vi "SetParametersAndor.vi"(6 "Error In":errorcluster, 8 "Camera Information":T7 {"VS Speed (us)" format="%.2f"}, 9 "Andor Initialization Error Codes":T6, 10 "Acquisition Parameters":T3={"Acquisition Mode"=enum."Single Scan", "Trigger Mode"=enum."Internal", "Frame \nTransfer"=FALSE, "Exposure Time (s)"=0.0, "Accumulation Cycle Time (s)"=0.0, "# Accumulations"=1, "# Kinetics"=1, "Kinetic Cycle Time (s)"=0.0, "Horizontal Bin Size"=1, "Vertical Bin Size"=1} {"Vertical Bin Size" min=1; "Horizontal Bin Size" min=1; "Kinetic Cycle Time (s)" format="%.2f"; "# Kinetics" min=1; "# Accumulations" min=1; "Accumulation Cycle Time (s)" format="%.2f"; "Exposure Time (s)" format="%.2f"}, 11 "Pre Initialized?":bool) -> (0 "error out":errorcluster, 2 "Calcualted Times":T1 {"Kinetic" format="%.4f"; "Accumulate" format="%.4f"; "Exposure" format="%.4f"}, 3 "Acq. Error Codes":T2)   [LabVIEW 2013]
uses:
  camera_information.ctl
  camera_controls.ctl
  <userlib>/atmcd32d.llb/AcquisitionMode_mode typedef.ctl
  <userlib>/atmcd32d.llb/TriggerMode_mode typedef.ctl
  set_parameters_states.ctl
  <userlib>/atmcd32d.llb/ReadMode_mode typedef.ctl
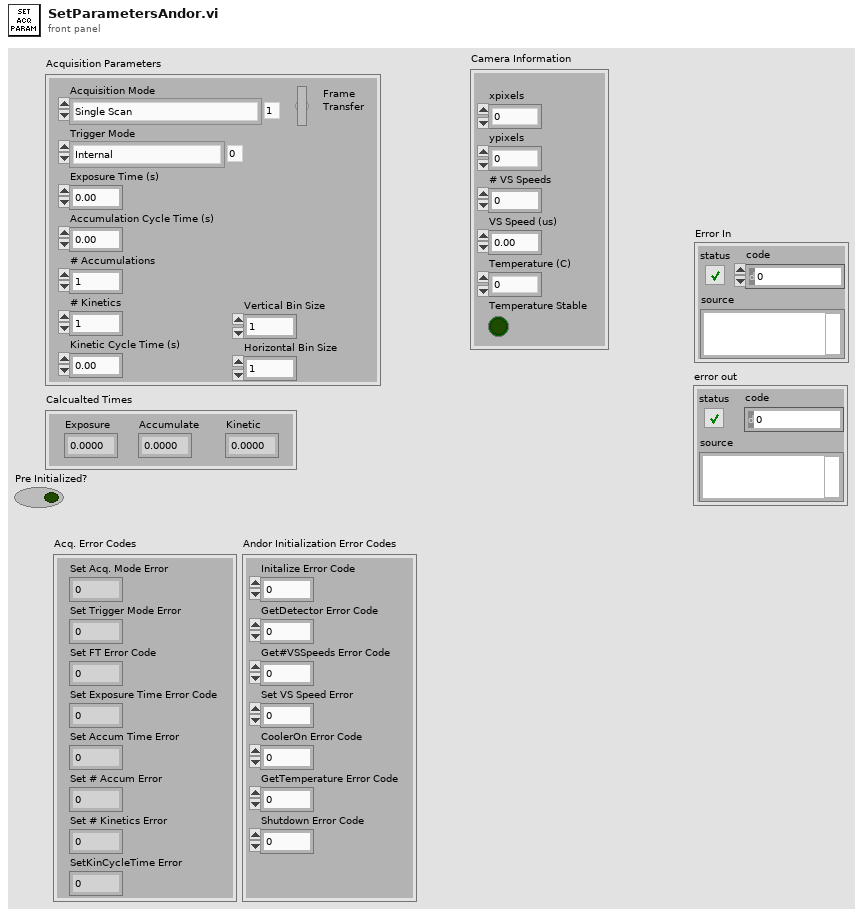
[diagram p1: front panel]
types:
  T1 = cluster{"Exposure":sgl, "Accumulate":sgl, "Kinetic":sgl}
  T2 = cluster{"Set Acq. Mode Error":u32, "Set Trigger Mode Error":u32, "Set FT Error Code":u32, "Set Exposure Time Error Code":u32, "Set Accum Time Error":u32, "Set # Accum Error":u32, "Set # Kinetics Error":u32, "SetKinCycleTime Error":u32}
  T3 = typedef "camera_controls.ctl" = cluster{"Acquisition Mode":T4, "Trigger Mode":T5, "Frame \nTransfer":bool, "Exposure Time (s)":sgl, "Accumulation Cycle Time (s)":sgl, "# Accumulations":i32, "# Kinetics":i32, "Kinetic Cycle Time (s)":sgl, "Horizontal Bin Size":i32, "Vertical Bin Size":i32}
  T4 = typedef "AcquisitionMode_mode typedef.ctl" = enum16{"Reserved (0)", "Single Scan", "Accumulate", "Kinetics", "Fast Kinetics", "Run Till Abort", "Reserved (6)", "Reserved (7)", "Reserved (8)", "Time Delayed Integration"}
  T5 = typedef "TriggerMode_mode typedef.ctl" = enum16{"Internal", "External", "N/A (2)", "N/A (3)", "N/A (4)", "N/A (5)", "External Start", "External Exposure (Bulb)", "N/A (8)", "External FVB EM", "Software", "N/A (11)", "External Charge Shifting"}
  T6 = cluster{"Initalize Error Code":u32, "GetDetector Error Code":u32, "Get#VSSpeeds Error Code":u32, "Set VS Speed Error":u32, "CoolerOn Error Code":u32, "GetTemperature Error Code":u32, "Shutdown Error Code":u32}
  T7 = typedef "camera_information.ctl" = cluster{"xpixels":i32, "ypixels":i32, "# VS Speeds":i32, "VS Speed (us)":sgl, "Temperature Stable":bool, "Temperature (C)":i32}
  T8 = typedef "set_parameters_states.ctl" = enum16{"Initialize", "Set Acq. Parameters", "Set Acq. Parameters 2", "Calculate", "Close Without Error", "Shutdown"}
  T9 = typedef "ReadMode_mode typedef.ctl" = enum16{"Full Vertical Binning", "Multi-Track", "Random-Track", "Single-Track", "Image"}
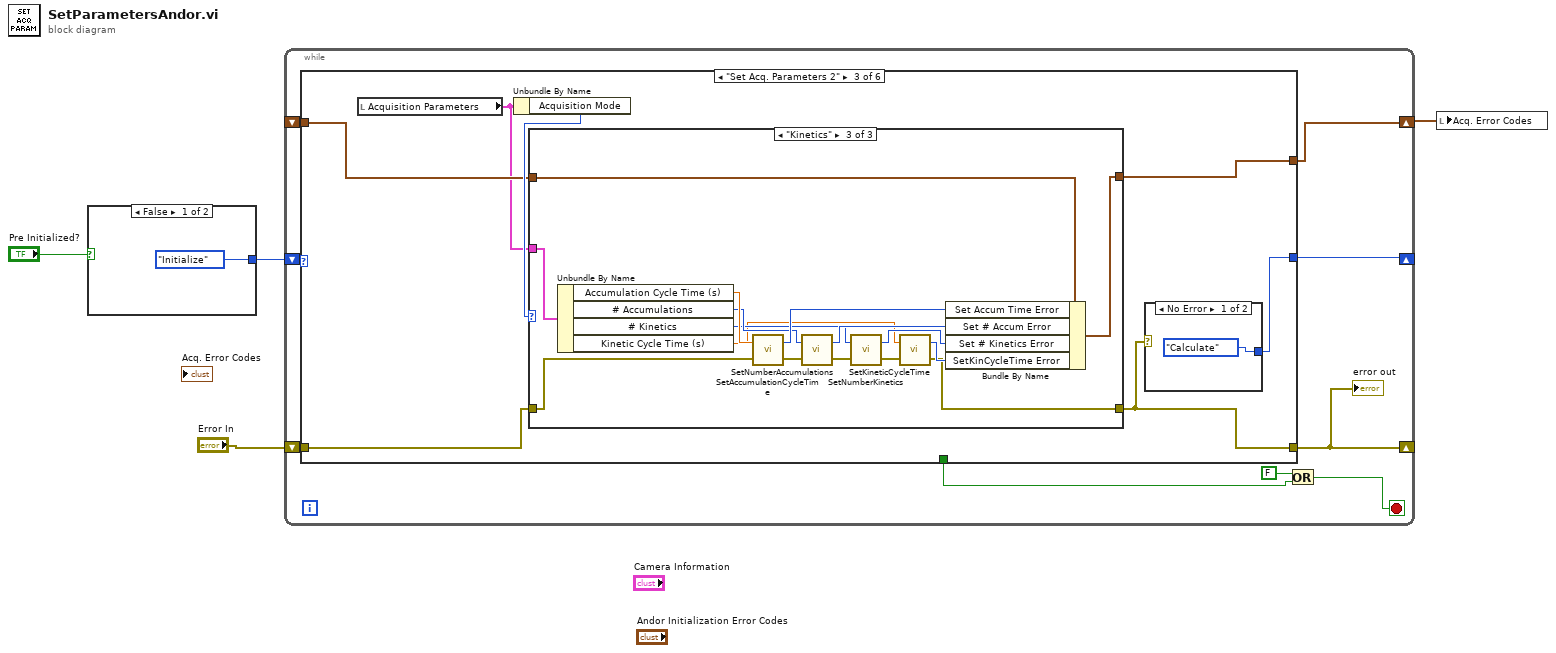
[diagram p0: block diagram]
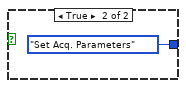
[diagram p2: hidden frame]
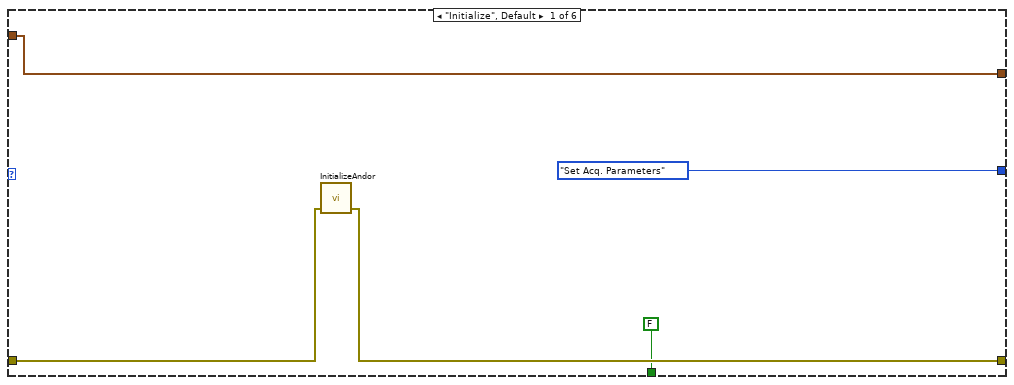
[diagram p3: hidden frame]
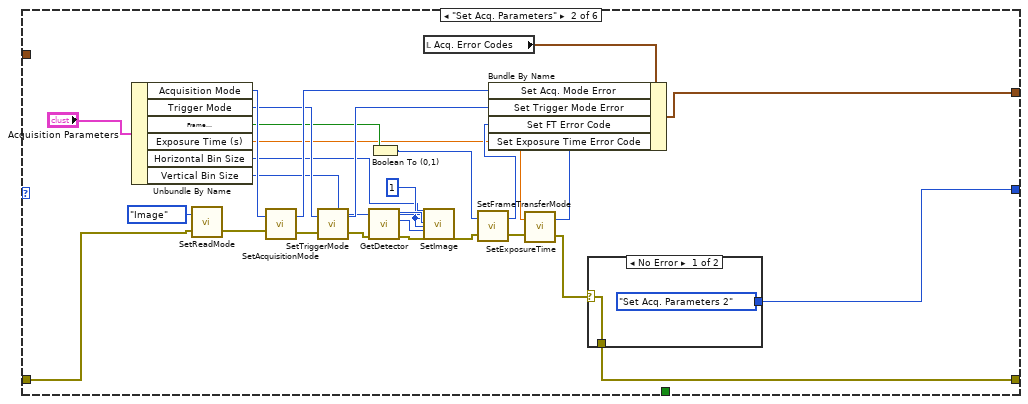
[diagram p4: hidden frame]
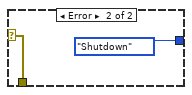
[diagram p5: hidden frame]
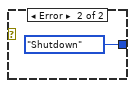
[diagram p6: hidden frame]
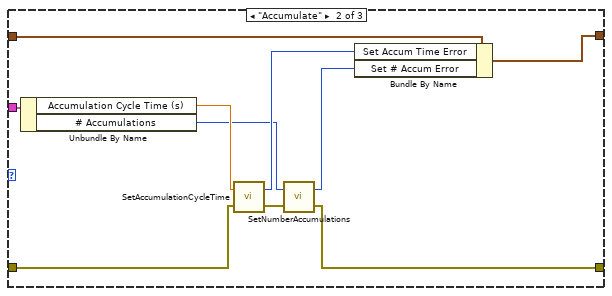
[diagram p8: hidden frame]
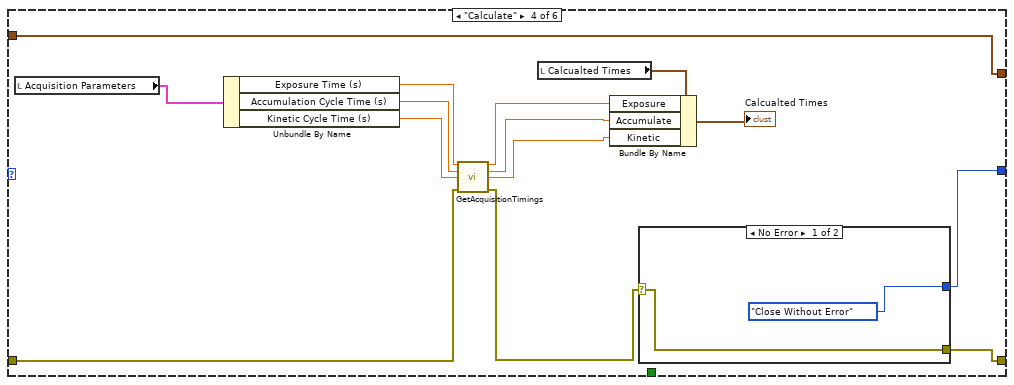
[diagram p9: hidden frame]
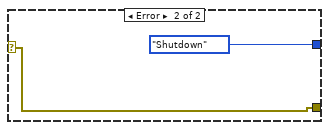
[diagram p10: hidden frame]
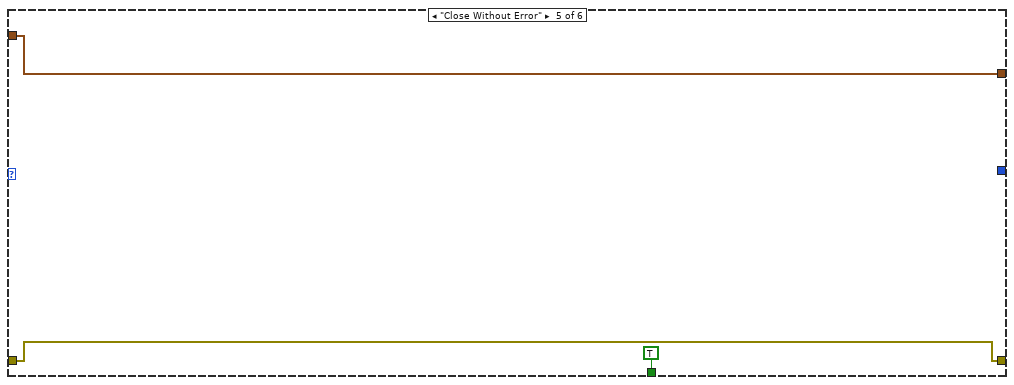
[diagram p11: hidden frame]
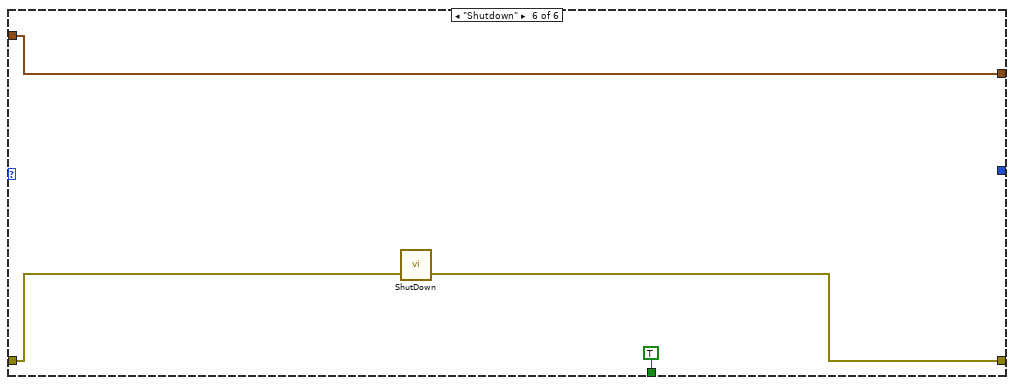
[diagram p12: hidden frame]
diagram:
  n1 = case shown="False" "Pre Initialized?" {
    tunnel: [set_parameters_states."Initialize" set_parameters_states."Set Acq. Parameters"] -> w4
    frame False {
    }
    frame True {
    }
  }
  n2 = while {
    shift-right: [w11] -> _
    shift-left: "Error In" -> [w14]
    shift-right: [w13] -> _
    shift-left: w4 -> [w15]
    shift-right: [w12] -> w2
    shift-left: _ -> [w7]
    stop <- w10 stop-if-true
    n3 = case shown="\"Set Acq. Parameters 2\"" w15 {
      tunnel: w14 -> [w20 w24 w58 w103 w109 w114]
      tunnel: [w19 w27 w54 w92 w109 w113] -> w11
      tunnel: [set_parameters_states."Set Acq. Parameters" w26 w53 w91 _ _] -> w13
      tunnel: [w16 w46 w55 w90 w108 w111] -> w12
      tunnel: [FALSE _ _ _ TRUE TRUE] -> w9
      tunnel: w7 -> [w16 _ w57 w90 w108 w111]
      frame "Initialize", Default {
        n4 = call "InitializeAndor.vi"("Error In"=w20) -> ("error out"=w19:errorcluster)  [unwired: 2 in, 2 out]
      }
      frame "Set Acq. Parameters" {
        w38 = 1
        n5 = Unbundle By Name("Acquisition Parameters") -> ("Acquisition Mode"=w44:T4, "Trigger Mode"=w42:T5, "Frame \nTransfer"=w34:bool, "Exposure Time (s)"=w31:sgl, "Horizontal Bin Size"=w21:i32, "Vertical Bin Size"=w22:i32)
        n6 = call <userlib>:"SetReadMode.vi"("error in (no error)"=w24, "mode"=ReadMode_mode_typedef."Image") -> ("error out"=w25:errorcluster)  [unwired: 1 out]
        n7 = call <userlib>:"SetAcquisitionMode.vi"("error in (no error)"=w25, "mode"=w44) -> ("error out"=w43:errorcluster, "DLL error code"=w47:u32)
        n8 = call <userlib>:"SetTriggerMode.vi"("error in (no error)"=w43, "mode"=w42) -> ("error out"=w36:errorcluster, "DLL error code"=w41:u32)
        n9 = call <userlib>:"GetDetector.vi"("error in (no error)"=w36) -> ("error out"=w40:errorcluster, "ypixels"=w37:i32, "xpixels"=w39:i32)  [unwired: 3 in, 1 out]
        n10 = Boolean To (0,1)(Boolean=w34) -> (0, 1=w33:i16)
        n11 = local read "Acq. Error Codes"() -> (w48:T2)
        n12 = call "SetImage.vi"("hbin"=w21, "vbin"=w22, "hstart"=w38, "hend"=w39, "vstart"=w38, "vend"=w37, "error in (no error)"=w40) -> ("error out"=w35:errorcluster)  [unwired: 19 in, 1 out]
        n13 = call <userlib>:"SetFrameTransferMode.vi"("error in (no error)"=w35, "mode"=w33) -> ("error out"=w29:errorcluster, "DLL error code"=w32:u32)
        n14 = call <userlib>:"SetExposureTime.vi"("error in (no error)"=w29, "time"=w31) -> ("error out"=w28:errorcluster, "DLL error code"=w30:u32)
        n15 = Bundle By Name(cluster=w48, "Set Acq. Mode Error"=w47, "Set Trigger Mode Error"=w41, "Set FT Error Code"=w32, "Set Exposure Time Error Code"=w30) -> (w46:T2)
        n16 = case shown="No Error" w28 {
          selector: w28 -> [w50 w51]
          tunnel: [w50 w51] -> w27
          tunnel: [set_parameters_states."Set Acq. Parameters 2" set_parameters_states."Shutdown"] -> w26
          frame No Error {
          }
          frame Error {
          }
        }
      }
      frame "Set Acq. Parameters 2" {
        n17 = local read "Acquisition Parameters"() -> (w56:T3)
        n18 = Unbundle By Name(w56) -> ("Acquisition Mode"=w59:T4)
        n19 = case shown="\"Kinetics\"" w59 {
          tunnel: [w63 w64 w74] -> w54
          tunnel: w58 -> [w63 w73 w89]
          tunnel: w57 -> [w62 w70 w87]
          tunnel: w56 -> [_ w72 w83]
          tunnel: [w62 w68 w84] -> w55
          frame "Single Scan", Default {
          }
          frame "Accumulate" {
            n20 = Unbundle By Name(w72) -> ("Accumulation Cycle Time (s)"=w71:sgl, "# Accumulations"=w66:i32)
            n21 = call <userlib>:"SetAccumulationCycleTime.vi"("error in (no error)"=w73, "time"=w71) -> ("error out"=w67:errorcluster, "DLL error code"=w69:u32)
            n22 = call <userlib>:"SetNumberAccumulations.vi"("error in (no error)"=w67, "number"=w66) -> ("error out"=w64:errorcluster, "DLL error code"=w65:u32)
            n23 = Bundle By Name(cluster=w70, "Set Accum Time Error"=w69, "Set # Accum Error"=w65) -> (w68:T2)
          }
          frame "Kinetics" {
            n24 = Unbundle By Name(w83) -> ("Accumulation Cycle Time (s)"=w82:sgl, "# Accumulations"=w81:i32, "# Kinetics"=w78:i32, "Kinetic Cycle Time (s)"=w76:sgl)
            n25 = call <userlib>:"SetAccumulationCycleTime.vi"("error in (no error)"=w89, "time"=w82) -> ("error out"=w88:errorcluster, "DLL error code"=w86:u32)
            n26 = call <userlib>:"SetNumberAccumulations.vi"("error in (no error)"=w88, "number"=w81) -> ("error out"=w80:errorcluster, "DLL error code"=w85:u32)
            n27 = call <userlib>:"SetNumberKinetics.vi"("error in (no error)"=w80, "number"=w78) -> ("error out"=w77:errorcluster, "DLL error code"=w79:u32)
            n28 = call <userlib>:"SetKineticCycleTime.vi"("error in (no error)"=w77, "time"=w76) -> ("error out"=w74:errorcluster, "DLL error code"=w75:u32)
            n29 = Bundle By Name(cluster=w87, "Set Accum Time Error"=w86, "Set # Accum Error"=w85, "Set # Kinetics Error"=w79, "SetKinCycleTime Error"=w75) -> (w84:T2)
          }
        }
        n30 = case shown="No Error" w54 {
          tunnel: [set_parameters_states."Calculate" set_parameters_states."Shutdown"] -> w53
          frame No Error {
          }
          frame Error {
          }
        }
      }
      frame "Calculate" {
        n31 = local read "Acquisition Parameters"() -> (w102:T3)
        n32 = Unbundle By Name(w102) -> ("Exposure Time (s)"=w101:sgl, "Accumulation Cycle Time (s)"=w100:sgl, "Kinetic Cycle Time (s)"=w99:sgl)
        n33 = call <userlib>:"GetAcquisitionTimings.vi"("exposure input"=w101, "accumulate input"=w100, "kinetic input"=w99, "error in (no error)"=w103) -> ("exposure"=w97:sgl, "accumulate"=w96:sgl, "kinetic"=w95:sgl, "error out"=w93:errorcluster)  [unwired: 7 in, 1 out]
        n34 = local read "Calcualted Times"() -> (w98:T1)
        n35 = Bundle By Name(cluster=w98, "Exposure"=w97, "Accumulate"=w96, "Kinetic"=w95) -> (→"Calcualted Times":T1)
        n36 = case shown="No Error" w93 {
          selector: w93 -> [w105 w106]
          tunnel: [w105 w106] -> w92
          tunnel: [set_parameters_states."Close Without Error" set_parameters_states."Shutdown"] -> w91
          frame No Error {
          }
          frame Error {
          }
        }
      }
      frame "Close Without Error" {
      }
      frame "Shutdown" {
        n37 = call <userlib>:"ShutDown.vi"("error in (no error)"=w114) -> ("error out"=w113:errorcluster)  [unwired: 1 in, 1 out]
      }
    }
    "error out" <- w11
    n38 = Or(x=FALSE, y=w9) -> (x .or. y?=w10:bool)
  }
  n39 = local write "Acq. Error Codes"(w2) -> ()
